vi "save_settings.vi"(3 "error in":errorcluster, 4 "settings_clus_file":T1={"CollectionInfoArray"=[{"Type"="Signal and Background", "LaserWave1"=249.7, "Shutter1"=TRUE, "LaserWave2"=0.0, "Shutter2"=FALSE, "FileEnd"="_SignalBack", "Collect"=TRUE}], "Delay scan"=FALSE, "channel enabled"=FALSE, "accurate scan"=FALSE, "update"=FALSE, "collection time"=0, "Wavelength Scan"=FALSE}, 5 "Path":path) -> (0 "error out":errorcluster, 2 "Pathout":path)   [LabVIEW 2019]
doc: "Takes the settings cluster and saves it as a xml file"
uses:
  Type defs/settings_file_ctrl.ctl
  Type defs/FileAcq_v1_Ctrl.ctl
  <vilib>/NI/GXML/GXML.lvlib
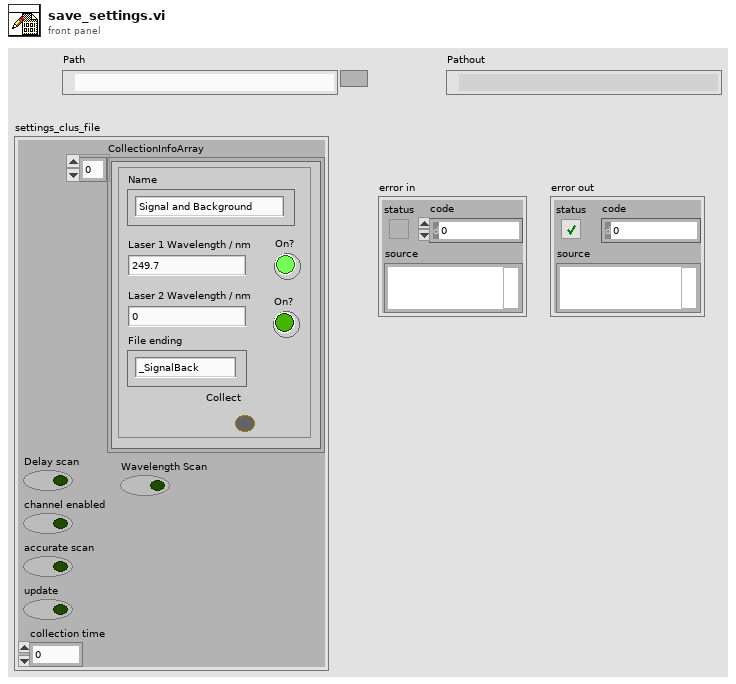
[diagram p1: front panel]
types:
  T1 = typedef "settings_file_ctrl.ctl" = cluster{"CollectionInfoArray":T2[], "Delay scan":bool, "channel enabled":bool, "accurate scan":bool, "update":bool, "collection time":i32, "Wavelength Scan":bool}
  T2 = typedef "FileAcq_v1_Ctrl.ctl" = cluster{"Type":string, "LaserWave1":dbl, "Shutter1":bool, "LaserWave2":dbl, "Shutter2":bool, "FileEnd":string, "Collect":bool}
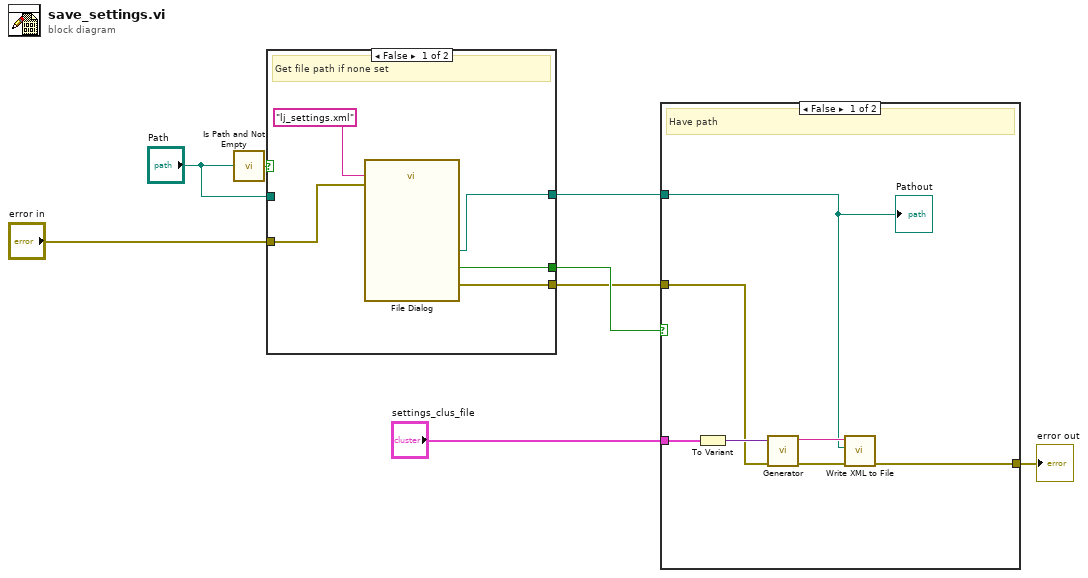
[diagram p0: block diagram]
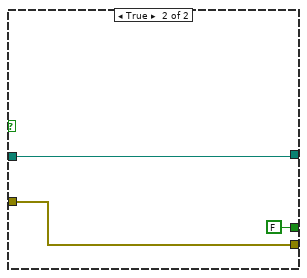
[diagram p3: hidden frame]
diagram:
  n1 = call <vilib>:"Is Path and Not Empty.vi"("path"="Path") -> ("Is Path and Not Empty?"=w8:bool)  [unwired: 4 in]
  n2 = case shown="False" w8 {
    tunnel: [w11 w16] -> w3
    tunnel: "Path" -> [_ w16]
    tunnel: [w13 w15] -> w4
    tunnel: "error in" -> [w12 w15]
    tunnel: [w10 FALSE ("cancelled")] -> w5
    frame False {
      # "Get file path if none set"
      n3 = call "File Dialog"("default name"="lj_settings.xml", "error in"=w12) -> ("selected path"=w11:path, "cancelled"=w10:bool, "error out"=w13:errorcluster)  [unwired: 10 in, 1 out]
    }
    frame True {
    }
  }
  n4 = case shown="False" w5 {
    tunnel: w4 -> [w21 w24]
    tunnel: w3 -> [w17 _]
    tunnel: [w18 w24] -> w2
    tunnel: "settings_clus_file" -> [w23 _]
    frame False {
      # "Have path"
      n5 = To Variant(anything=w23) -> (Variant=w22:variant)
      n6 = call <vilib>:"Generator.vi"("error in"=w21, "Variant"=w22) -> ("error out"=w20:errorcluster, "XML String Out"=w19:string)  [unwired: 8 in]
      n7 = call <vilib>:"Write XML to File.vi"("error in"=w20, "XML File Path"=w17, "XML Input"=w19) -> ("error out"=w18:errorcluster)  [unwired: 8 in]
      "Pathout" <- w17
    }
    frame True {
      # "Cancelled so still no path"
    }
  }
  "error out" <- w2
